vi "Write Value.vi"(8 "error in (no error)":errorcluster, 10 "Value":string, 11 "Setting in":refnum<class "Setting.lvclass">) -> (0 "error out":errorcluster, 3 "Setting out":refnum<class "Setting.lvclass">)   [LabVIEW 2023, in "HAF.lvlib" / "Setting.lvclass"]
doc: "Saves a new Value for the Setting."
uses:
  Setting.lvclass
  Setting.lvclass/Setting.ctl
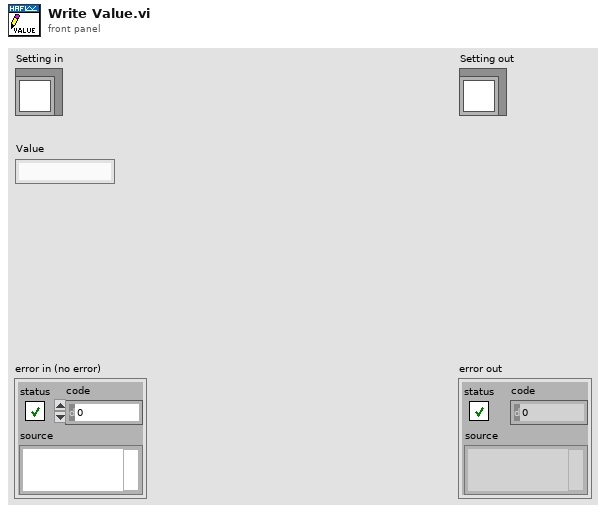
[diagram p1: front panel]
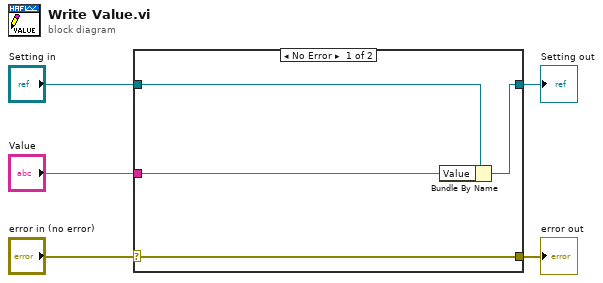
[diagram p0: block diagram]
diagram:
  n1 = case shown="No Error" "error in (no error)" {
    selector: "error in (no error)" -> [w9 w10]
    tunnel: [w9 w10] -> w4
    tunnel: [w7 w11] -> w2
    tunnel: "Setting in" -> [w8 w11]
    tunnel: "Value" -> [w6 _]
    frame No Error {
      n2 = Bundle By Name(cluster=w8, "Value"=w6) -> (w7:refnum<class "Setting.lvclass">)
    }
    frame Error {
    }
  }
  "error out" <- w4
  "Setting out" <- w2
